vi "xBoxTriggerButtonOp.vi"(11 "zAxis":dbl) -> (1 "Throw":bool, 3 "Lob":bool)   [LabVIEW 2014]
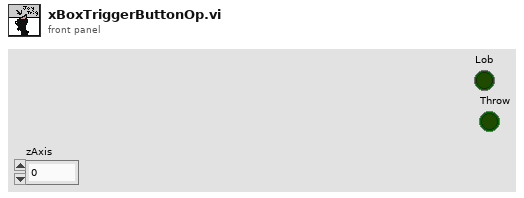
[diagram p1: front panel]
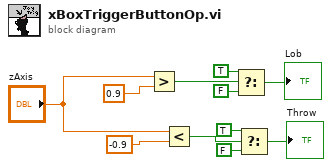
[diagram p0: block diagram]
diagram:
  n1 = Greater?(x="zAxis", y=0.9) -> (0:w5:bool)
  n2 = Less?(x="zAxis", y=-0.9) -> (x < y?=w1:bool)
  n3 = Select(t=TRUE, s=w5, f=FALSE) -> (s? t:f=→"Lob":bool)
  n4 = Select(t=TRUE, s=w1, f=FALSE) -> (s? t:f=→"Throw":bool)
